vi "Modell Beschleunigung Sub.vi"(6 "Masse (Pendel)":dbl, 9 "Pendellänge":dbl, 10 "Beschleunigung":dbl, 11 "Trägheitsmoment (Pendel)":dbl) -> (1 "Winkelgeschw.":dbl, 2 "Position":dbl, 3 "Geschwindigkeit":dbl, 4 "Winkel":dbl)   [LabVIEW 2013]
uses:
  <vilib>/Simulation/Implementation/Shared/SIMSCR Execution Mode.ctl
  <vilib>/Simulation/Scripting/Companion Diagram/SimConfigNode/SimParams.ctl
  <vilib>/Simulation/Scripting/Companion Diagram/SimConfigNode/_simSolvers.ctl
  <vilib>/Simulation/Param Hierarchy/Typedefs/SIMPH Param Control Actions.ctl
  <vilib>/Simulation/Implementation/Shared/SIM limit type.ctl
  <vilib>/Simulation/Implementation/Shared/NILVSim_ParamChanged.vi
  <vilib>/Simulation/Implementation/Shared/NILVSIM_BeginStep.vi
  <vilib>/Simulation/ContinuousLinear/Implementation/NILVSim Integrator new.llb/SIM Integrator distributor (scalar).vi
  <vilib>/Simulation/SignalArithmetic/Implementation/NILVSim Gain.llb/SIM Gain (scalar).vi
  <vilib>/Simulation/ContinuousLinear/Implementation/NILVSim Integrator new.llb/SIM Integrator collector (scalar).vi
  <vilib>/Simulation/Implementation/Shared/NILVSim_Manager.vi
  <vilib>/Simulation/Implementation/Shared/NILVSim_FinalizeModel.vi
  <vilib>/Simulation/Implementation/Shared/SIM Unbundle Sim Info.vi
  <vilib>/Utility/error.llb/Clear Errors.vi
  <vilib>/Simulation/Implementation/Shared/NILVSim_GetModelError.vi
  <vilib>/Simulation/Implementation/Shared/SIM SimErrorHandler.vi
  <vilib>/Simulation/Implementation/Shared/SIM Bundle Sim Info.vi
  <vilib>/Simulation/Implementation/Shared/SIMSH Read Queue.vi
  <vilib>/Simulation/Implementation/Shared/NILVSim_Initialize.vi
  <vilib>/Simulation/Utility/Implementation/NILVSim Get Time and IsAcceptedStep.vi
  <vilib>/Simulation/Scripting/Companion Diagram/SimConfigNode/SimDog.xnode
  <vilib>/Simulation/Implementation/XNodeFramework/SimXNode/SimX.xnode
  <vilib>/Simulation/ContinuousLinear/Implementation/NILVSim Integrator new.llb/SIM Integrator (scalar).vi
  <vilib>/Simulation/Implementation/Shared/NI_SIM_Implementation.lvlib
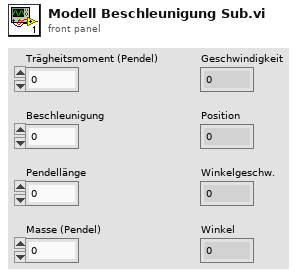
[diagram p1: front panel]
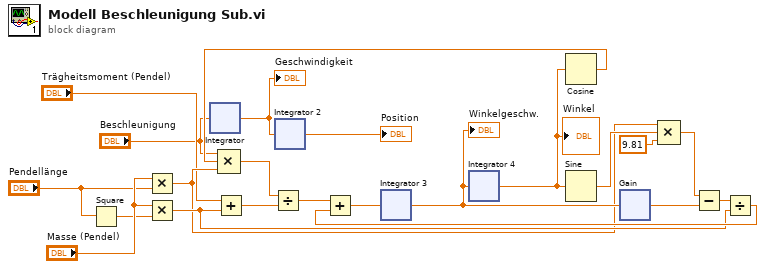
[diagram p0: block diagram]
diagram:
  n1 = Square ("Quadrat")(x="Pendellänge") -> (x^2=w7:dbl)
  n2 = Multiply ("Multiplizieren")(x="Masse (Pendel)", y="Pendellänge") -> (x*y=w11:dbl)
  n3 = Multiply ("Multiplizieren 2")(x="Masse (Pendel)", y=w7) -> (x*y=w16:dbl)
  n4 = xnode "Integrator"("input"="Beschleunigung") -> ("output"=w1:dbl)  [unwired: 9 in, 2 out]
  "Geschwindigkeit" <- w1
  n5 = Add ("Addieren")(x="Trägheitsmoment (Pendel)", y=w16) -> (x+y=w10:dbl)
  n6 = xnode "Integrator 2"("input"=w1) -> ("output"=→"Position":dbl)  [unwired: 9 in, 2 out]
  n7 = Compound Arithmetic op=MULTIPLY ("Mehrfacharithmetik")("Beschleunigung", w5, w11) -> (w3:dbl)
  n8 = Divide ("Dividieren")(x=w3, y=w10) -> (x/y=w18:dbl)
  n9 = Add ("Addieren 2")(x=w18, y=w17) -> (x+y=w19:dbl)
  n10 = xnode "Integrator 3"("input"=w19) -> ("output"=w22:dbl)  [unwired: 9 in, 2 out]
  "Winkelgeschw." <- w22
  n11 = xnode "Integrator 4"("input"=w22) -> ("output"=w21:dbl)  [unwired: 9 in, 2 out]
  "Winkel" <- w21
  n12 = Cosine ("Cosinus")(x=w21) -> (cos(x)=w5:dbl)
  n13 = Sine ("Sinus")(x=w21) -> (sin(x)=w12:dbl)
  n14 = xnode "Gain"("input"=w22) -> ("output"=w20:dbl)  [unwired: 3 in]
  n15 = Compound Arithmetic op=MULTIPLY ("Mehrfacharithmetik 2")(w11, w12, 9.81 ("Wert")) -> (w14:dbl)
  n16 = Subtract ("Subtrahieren")(x=w14, y=w20) -> (x-y=w15:dbl)
  n17 = Divide ("Dividieren 3")(x=w15, y=w16) -> (x/y=w17:dbl)
